vi "Dequeue-Pop Element.vi"(8 "error in":errorcluster, 9 "error if not found?":bool=TRUE caption="error if not found? (T)", 11 "Buffer in":refnum<data-value>) -> (0 "error out":errorcluster, 1 "found":bool, 2 "element":variant, 3 "Buffer":refnum<data-value>, 4 "buffer empty?":bool)   [LabVIEW 2013, in "CircularBuffer.lvlib" / "VariantBuffer.lvclass"]
doc: "This VI is a definition for future."
uses:
  VariantBuffer.lvclass
  VariantBuffer.lvclass/VariantBuffer.ctl
  buffer-errors -- ring.ctl
  buffer-event -- enum.ctl
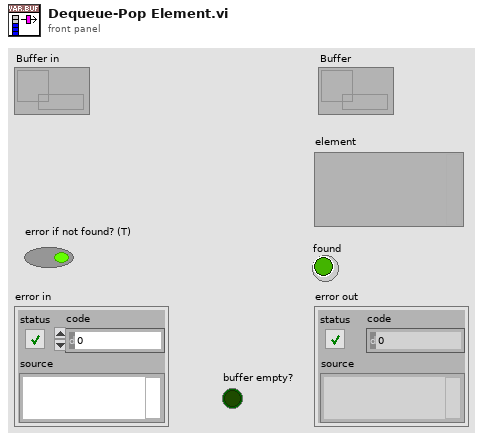
[diagram p1: front panel]
types:
  T1 = typedef "CircularBuffer.lvlib/VariantBuffer.lvclass/buffer-type -- enum.ctl" = enum16{"Queue", "Stack"}
  T2 = typedef "CircularBuffer.lvlib/VariantBuffer.lvclass/buffer-errors -- ring.ctl" = i32
  T3 = typedef "CircularBuffer.lvlib/VariantBuffer.lvclass/buffer-event -- enum.ctl" = enum16{"element-added", "element-removed", "filled", "emptied", "resized", "default-changed", "destroyed"}
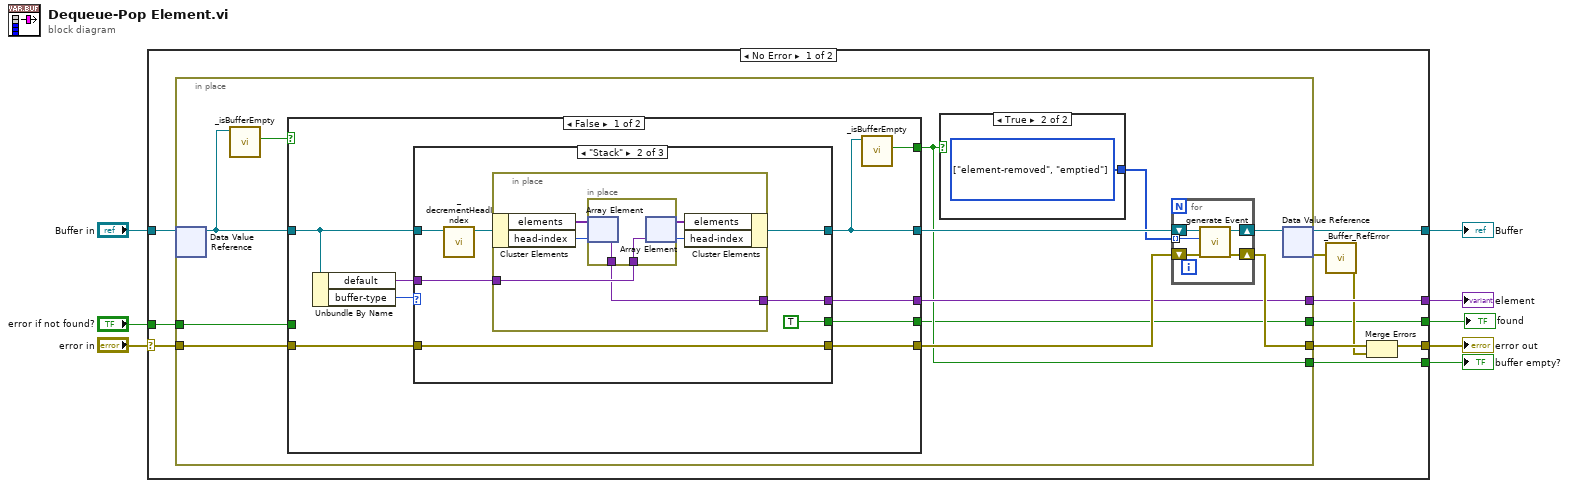
[diagram p0: block diagram]
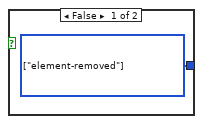
[diagram p2: hidden frame]
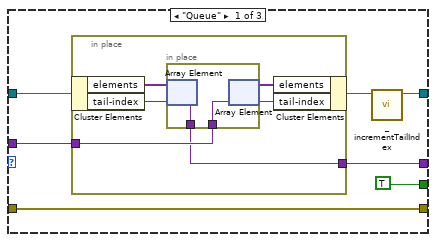
[diagram p3: hidden frame]
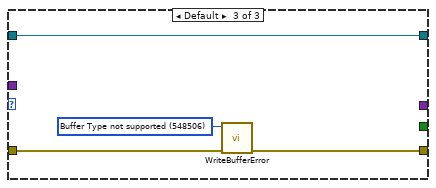
[diagram p4: hidden frame]
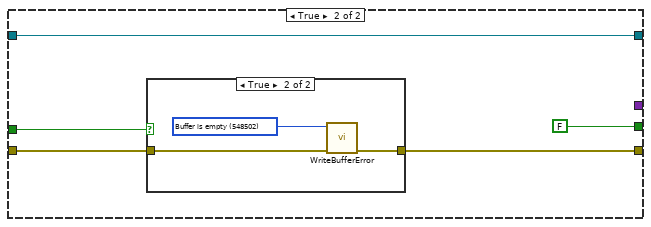
[diagram p5: hidden frame]
diagram:
  n1 = case shown="No Error" "error in" {
    selector: "error in" -> [w17 w92]
    tunnel: "Buffer in" -> [w19 w91]
    tunnel: [w15 w91] -> w7
    tunnel: [w18 w92] -> w6
    tunnel: [w14 _] -> w4
    tunnel: [w13 _] -> w3
    tunnel: [w10 _] -> w2
    tunnel: "error if not found?" -> [w9 _]
    frame No Error {
      n2 = in-place {
        in-place-border: w17 -> [w29]
        in-place-border: [w26] -> w16
        in-place-border: [w23] -> w14
        in-place-border: [w22] -> w13
        in-place-border: [w21] -> w10
        in-place-border: w9 -> [w20]
        n3 = in-place-dvr #1(w19) -> (w31:refnum<class "VariantBuffer.lvclass">)  [unwired: 1 out]
        n4 = call "_isBufferEmpty.vi"("VariantBuffer in"=w31) -> ("isEmpty"=w30:bool)  [unwired: 10 in]
        n5 = case shown="False" w30 {
          tunnel: [w47 w84] -> w27
          tunnel: [w46 _] -> w22
          tunnel: w31 -> [w45 w84]
          tunnel: w29 -> [w43 w86]
          tunnel: [w42 w85] -> w25
          tunnel: [w40 _] -> w23
          tunnel: [w39 FALSE] -> w21
          tunnel: w20 -> [_ w82]
          frame False {
            n6 = Unbundle By Name(w45) -> ("default"=w41:variant, "buffer-type"=w44:T1)
            n7 = case shown="\"Stack\"" w44 {
              tunnel: [w50 w66 w81] -> w47
              tunnel: w45 -> [w49 w65 w81]
              tunnel: w43 -> [w54 w69 w80]
              tunnel: [w54 w69 w79] -> w42
              tunnel: w41 -> [w53 w68 _]
              tunnel: [w52 w67 _] -> w40
              tunnel: [TRUE TRUE _] -> w39
              frame "Queue" {
                n8 = in-place {
                  in-place-border: w53 -> [w56]
                  in-place-border: [w55] -> w52
                  n9 = in-place-cluster #2(w49) -> ("elements"=w60:variant[], "tail-index"=w58:i32)
                  n10 = in-place {
                    in-place-border: w56 -> [w62]
                    in-place-border: [w61] -> w55
                    n11 = in-place-array #3(w60, w58) -> (w61:variant)
                    n12 = in-place-array #3(w62) -> (w59:variant[], w57:i32)
                  }
                  n13 = in-place-cluster #2("elements"=w59, "tail-index"=w57) -> (w51:refnum<class "VariantBuffer.lvclass">)
                }
                n14 = call "_incrementTailIndex.vi"("VariantBuffer in"=w51) -> ("VariantBuffer out"=w50:refnum<class "VariantBuffer.lvclass">)  [unwired: 10 in]
              }
              frame "Stack" {
                n15 = call "_decrementHeadIndex.vi"("VariantBuffer in"=w65) -> ("VariantBuffer out"=w64:refnum<class "VariantBuffer.lvclass">)  [unwired: 10 in]
                n16 = in-place {
                  in-place-border: w68 -> [w71]
                  in-place-border: [w70] -> w67
                  n17 = in-place-cluster #4(w64) -> ("elements"=w75:variant[], "head-index"=w73:i32)
                  n18 = in-place {
                    in-place-border: w71 -> [w77]
                    in-place-border: [w76] -> w70
                    n19 = in-place-array #5(w75, w73) -> (w76:variant)
                    n20 = in-place-array #5(w77) -> (w74:variant[], w72:i32)
                  }
                  n21 = in-place-cluster #4("elements"=w74, "head-index"=w72) -> (w66:refnum<class "VariantBuffer.lvclass">)
                }
              }
              frame Default {
                w78 = T2 548506 items=["No error"=0, "Generic Buffer error"=548500, "Buffer is full"=548501, "Buffer is empty"=548502, "Buffer size cannot be 0"=548503, "Buffer reference is invalid"=548504, "Buffer event reference invalid"=548505, "Buffer Type not supported"=548506] ("buffer-errors")
                n22 = call "WriteBufferError.vi"("error in (no error)"=w80, "buffer-errors"=w78) -> ("error out"=w79:errorcluster)  [unwired: 9 in]
              }
            }
            n23 = call "_isBufferEmpty.vi"("VariantBuffer in"=w47) -> ("isEmpty"=w46:bool)  [unwired: 10 in]
          }
          frame True {
            n24 = case shown="True" w82 {
              tunnel: w86 -> [w87 w90]
              tunnel: [w87 w88] -> w85
              frame False {
              }
              frame True {
                w89 = T2 548502 items=["No error"=0, "Generic Buffer error"=548500, "Buffer is full"=548501, "Buffer is empty"=548502, "Buffer size cannot be 0"=548503, "Buffer reference is invalid"=548504, "Buffer event reference invalid"=548505, "Buffer Type not supported"=548506] ("buffer-errors")
                n25 = call "WriteBufferError.vi"("error in (no error)"=w90, "buffer-errors"=w89) -> ("error out"=w88:errorcluster)  [unwired: 9 in]
              }
            }
          }
        }
        n26 = case shown="True" w22 {
          tunnel: [w32 w33] -> w24
          frame False {
            w32 = T3[] [enum."element-removed"] items=["element-added", "element-removed", "filled", "emptied", "resized", "default-changed", "destroyed"]
          }
          frame True {
            w33 = T3[] [enum."element-removed", enum."emptied"] items=["element-added", "element-removed", "filled", "emptied", "resized", "default-changed", "destroyed"]
          }
        }
        n27 = for {
          tunnel: w24 -> [w36] mode=indexing
          shift-right: [w38] -> w28
          shift-left: w27 -> [w37]
          shift-right: [w35] -> w26
          shift-left: w25 -> [w34]
          n28 = call "_generate Event.vi"("error in"=w34, "event"=w36, "VariantBuffer"=w37) -> ("error out"=w35:errorcluster, "VariantBuffer out"=w38:refnum<class "VariantBuffer.lvclass">)  [unwired: 7 in]
        }
        n29 = in-place-dvr #1(w28) -> (w15:refnum<data-value>, w12:errorcluster)
      }
      n30 = call "_Buffer_RefError.vi"("error in (no error)"=w12) -> ("error out"=w11:errorcluster)  [unwired: 10 in]
      n31 = Merge Errors(w16, w11) -> (w18:errorcluster)
    }
    frame Error {
    }
  }
  "error out" <- w6
  "Buffer" <- w7
  "element" <- w4
  "buffer empty?" <- w3
  "found" <- w2
